vi "test Add Duplicate Alias.vi"(8 "error in (no error)":errorcluster, 11 "TestCase in":refnum<class "Routing and Faulting Aliases Unit Tests.lvclass">) -> (0 "error out":errorcluster, 3 "TestCase out":refnum<class "Routing and Faulting Aliases Unit Tests.lvclass">)   [LabVIEW 2017, in "Routing and Faulting Aliases Unit Tests.lvclass"]
uses:
  Routing and Faulting Aliases Unit Tests.lvclass
  Shared/Alias Mapping.ctl
  System Explorer/Alias.ctl
  System Explorer/Endpoint.ctl
  Routing and Faulting Aliases Unit Tests.lvclass/Routing and Faulting Aliases Unit Tests.ctl
  <vilib>/addons/_JKI Toolkits/VI Tester/TestCase.llb/TestCase.lvclass
  System Explorer/Routing and Faulting System Explorer.lvlib
  Scripting/Routing and Faulting Scripting.lvlib
  Shared/Routing and Faulting Shared.lvlib
  C:/Program Files (x86)/National Instruments/LabVIEW 2017/vi.lib/addons/_JKI Toolkits/VI Tester/TestCase.llb/TestCase.lvclass
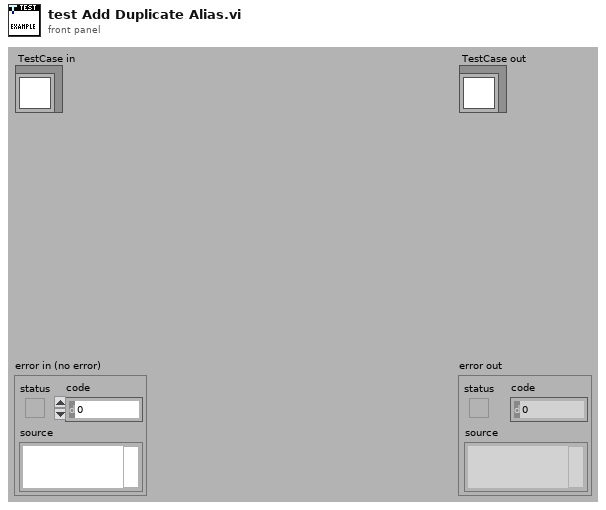
[diagram p1: front panel]
types:
  T1 = typedef "Routing and Faulting System Explorer.lvlib/Endpoint.ctl" = string
  T2 = typedef "Routing and Faulting Shared.lvlib/Alias Mapping.ctl" = cluster{"Endpoint":string, "Alias":string}
  T3 = typedef "Routing and Faulting System Explorer.lvlib/Alias.ctl" = cluster{"Endpoint":T1, "Alias":string, "Remove":bool}
  T4 = typedef "Custom Device API.lvlib/Custom Device Item Ref.ctl" = u64
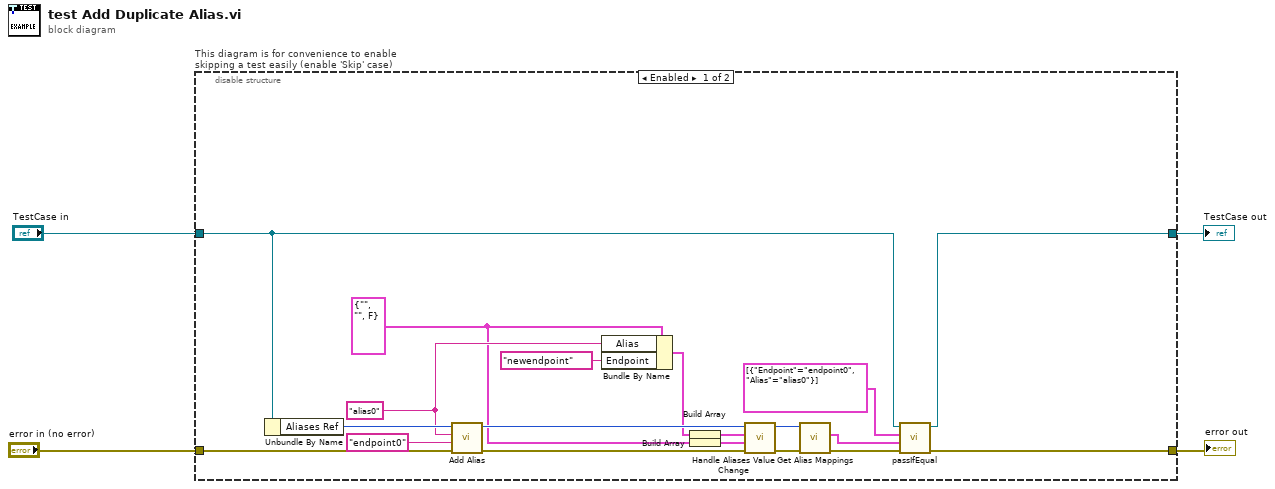
[diagram p0: block diagram]
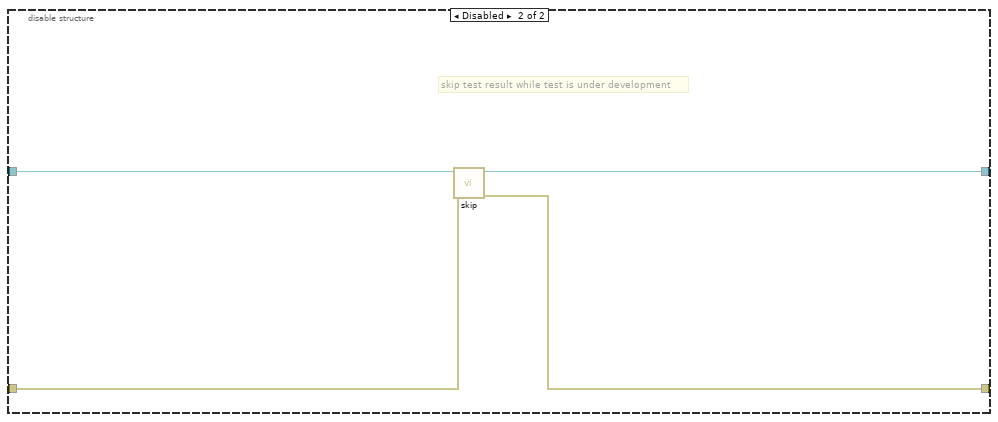
[diagram p2: hidden frame]
diagram:
  n1 = disable-structure "This diagram is for convenience to enable skipping a test easily (enable 'Skip' case)" shown="Enabled" {
    disable-tunnel: "TestCase in" -> [w17 w27]
    disable-tunnel: [w16 w25] -> w1
    disable-tunnel: [w20 w26] -> w3
    disable-tunnel: "error in (no error)" -> [w14 w24]
    frame Enabled {
      w5 = T3 {"Endpoint"="", "Alias"="", "Remove"=FALSE} ("Alias")
      w6 = "alias0" ("Alias")
      n2 = Unbundle By Name(w17) -> ("Aliases Ref"=w15:T4)
      n3 = call "Add Alias.vi"("error in (no error)"=w14, "Endpoint"="endpoint0", "Alias"=w6, "Endpoint Aliases Ref in"=w15) -> ("error out"=w12:errorcluster, "Endpoint Aliases Ref out"=w13:T4)  [unwired: 6 in]
      n4 = Bundle By Name(cluster=w5, "Alias"=w6, "Endpoint"=T1 "newendpoint") -> (w8:T3)
      n5 = Build Array(w8) -> (w9:T3[])
      n6 = Build Array(w5) -> (w10:T3[])
      n7 = call "Handle Aliases Value Change.vi"("error in (no error)"=w12, "OldVal"=w10, "NewVal"=w9, "Aliases Ref in"=w13) -> ("error out"=w23:errorcluster, "Aliases Ref out"=w22:T4)  [unwired: 6 in]
      n8 = call "Get Alias Mappings.vi"("error in (no error)"=w23, "Endpoint Aliases Ref in"=w22) -> ("error out"=w21:errorcluster, "Alias Mappings"=w19:T2[])  [unwired: 7 in, 1 out]
      n9 = call-dynamic "passIfEqual.vi"("error in (no error)"=w21, "y"=w19, "x"=T2[] [{"Endpoint"="endpoint0", "Alias"="alias0"}] ("Alias Mappings"), "TestCase in"=w17) -> ("error out"=w20:errorcluster, "TestCase out"=w16:refnum<class "Routing and Faulting Aliases Unit Tests.lvclass">)  [unwired: 6 in]
    }
    frame Disabled {
      # "skip test result while test is under development"
      n10 = call <vilib>:"skip.vi"("error in (no error)"=w24, "TestCase in"=w27) -> ("error out"=w26:errorcluster, "TestCase out"=w25:refnum<class "Routing and Faulting Aliases Unit Tests.lvclass">)  [unwired: 8 in]
    }
  }
  "error out" <- w3
  "TestCase out" <- w1
